vi "Configure Sense Voltage Up And Down.vi"(8 "error in (no error)":errorcluster, 9 "Voltage Value : 0":u32, 10 "Up&Down ( 0 : Up)":u16(ring) items=["Up", "Down"], 11 "VISA resource name":refnum<visa-resource-name>) -> (0 "error out":errorcluster, 3 "VISA resource name out":refnum<visa-resource-name>)   [LabVIEW 2015, in "IT8900A-E.lvlib"]
doc: "This command sets the voltage point at which the output voltage of the object to be measured rises and drops at the load.\n\n<b>Up&Down ( 0 : Up)</b>\n0: Up\n1: Down"
uses:
  <instrlib>/IT8900/IT8900A-E.lvlib
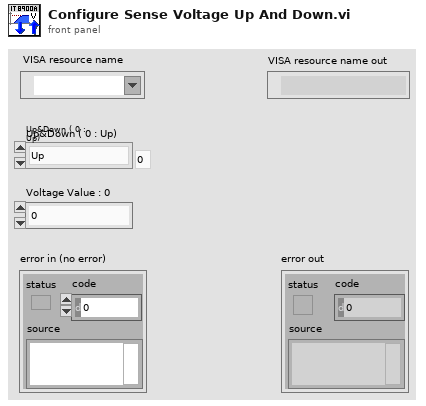
[diagram p1: front panel]
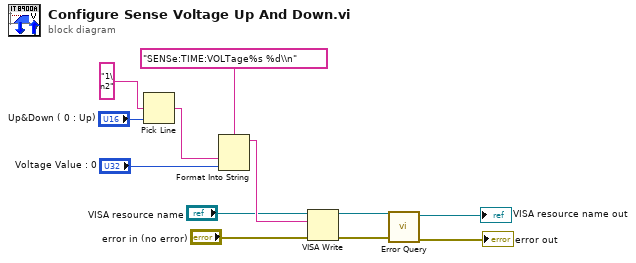
[diagram p0: block diagram]
diagram:
  n1 = Pick Line(multi-line string="1\n2", line index="Up&Down ( 0 : Up)") -> (output string=w1:string)  [unwired: 1 in]
  n2 = Format Into String(format string="SENSe:TIME:VOLTage%s %d\\n", w1, "Voltage Value : 0") -> (resulting string=w11:string)  [unwired: 2 in, 1 out]
  n3 = VISA Write(VISA resource name="VISA resource name", write buffer=w11, error in (no error)="error in (no error)") -> (VISA resource name out=w8:refnum<visa-resource-name>, error out=w6:errorcluster)  [unwired: 1 out]
  n4 = call <instrlib>:"Error Query.vi"("error in (no error)"=w6, "VISA resource name"=w8) -> ("error out"=→"error out":errorcluster, "VISA resource name out"=→"VISA resource name out":refnum<visa-resource-name>)  [unwired: 6 in, 2 out]
